vi "设置缓存有效.vi"(8 "error in (no error)":errorcluster caption="错误输入（无错误）", 11 "图形 输入":refnum<class "图形.lvclass"> caption="DNL_LabVIEW Object in") -> (0 "error out":errorcluster caption="错误输出", 3 "图形 输出":refnum<class "图形.lvclass"> caption="DNL_LabVIEW Object out")   [LabVIEW 2011, in "图形.lvclass"]
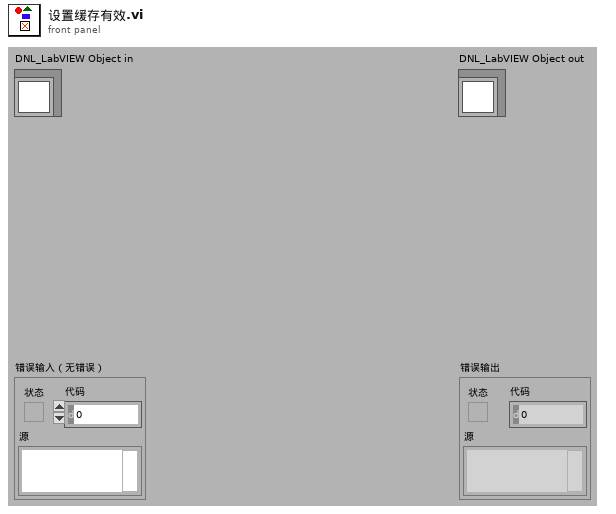
[diagram p1: front panel]
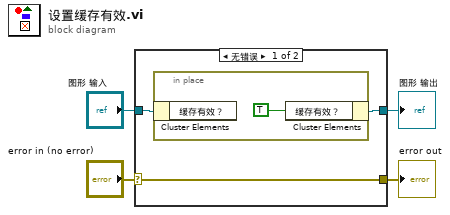
[diagram p0: block diagram]
diagram:
  n1 = case shown="无错误" "error in (no error)" {
    selector: "error in (no error)" -> [w7 w10]
    tunnel: [w7 w10] -> w3
    tunnel: [w5 w9] -> w1
    tunnel: "图形 输入" -> [w6 w9]
    frame No Error {
      n2 = in-place {
        n3 = in-place-cluster #1(w6) -> ()  [unwired: 1 out]
        n4 = in-place-cluster #1("缓存有效？"=TRUE) -> (w5:refnum<class "图形.lvclass">)
      }
    }
    frame Error {
    }
  }
  "error out" <- w3
  "图形 输出" <- w1
